vi "Assign DIO Bits to Execute Stored Program.vi"(4 "error in (no error)":errorcluster, 5 "Program Name":string, 6 "Bit Number (0)":i32 min=0 max=15, 7 "VISA resource name":refnum<visa-resource-name>) -> (0 "error out":errorcluster, 3 "VISA resource name out":refnum<visa-resource-name>)   [LabVIEW 2020, in "Newport ESP301.lvlib"]
doc: "This command is used to assign DIO bits for initiating the execution of a desired stored program. Execution of the stored program begins when the specified DIO bit changes its state from HIGH to LOW logic level.\n<B>NOTE:</B> Each DIO bit has a pulled-up resistor to +5V. Therefore, all bits will be at HIGH logic level if not connected to external circuit and configured as input."
uses:
  Newport ESP301.lvlib
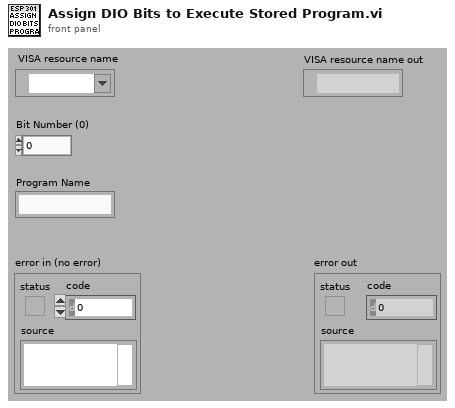
[diagram p1: front panel]
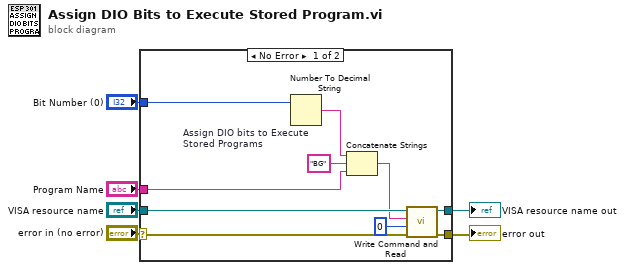
[diagram p0: block diagram]
diagram:
  n1 = case shown="No Error" "error in (no error)" {
    selector: "error in (no error)" -> [w10 w18]
    tunnel: [w8 w18] -> w6
    tunnel: "VISA resource name" -> [w13 w17]
    tunnel: [w9 w17] -> w5
    tunnel: "Bit Number (0)" -> [w14 _]
    tunnel: "Program Name" -> [w7 _]
    frame No Error {
      w16 = "BG"  # Assign DIO bits to Execute Stored Programs
      n2 = Number To Decimal String(number=w14) -> (decimal integer string=w15:string)  [unwired: 1 out]
      n3 = Concatenate Strings(w15, w16, w7) -> (w12:string)
      n4 = call "Write Command and Read.vi"("error in (no error)"=w10, "Bytes to read (100)"=u32 0, "Command"=w12, "VISA resource name"=w13) -> ("error out"=w8:errorcluster, "VISA resource name out"=w9:refnum<visa-resource-name>)  [unwired: 1 in, 3 out]
    }
    frame Error {
    }
  }
  "error out" <- w6
  "VISA resource name out" <- w5
